vi "orc-red-threshing.vi"(5 "Blue or Luma or Val or Inten Range":cluster{"Lower value":i32, "Upper value":i32}={"Lower value"=0, "Upper value"=255}, 7 "Green or Sat Range":cluster{"Lower value":i32, "Upper value":i32}={"Lower value"=93, "Upper value"=255}, 9 "Red or Hue Range":cluster{"Lower value":i32, "Upper value":i32}={"Lower value"=6, "Upper value"=11}, 10 "Cluster":cluster{"Min Radius":sgl, "Max Radius":sgl}={"Min Radius"=10.0, "Max Radius"=100.0}, 11 "Image Src":T2, 13 "error in (no error)":errorcluster) -> (0 "Image Out":T2(plugin-control), 4 "Circles Data (calibrated)":T1(array[cluster]), 8 "Nb Circles":i32, 15 "error out":errorcluster)   [LabVIEW 2009]
uses:
  <vilib>/vision/Image Controls.llb/IMAQ Image.ctl
  <vilib>/vision/NI_Vision_Development_Module.lvlib
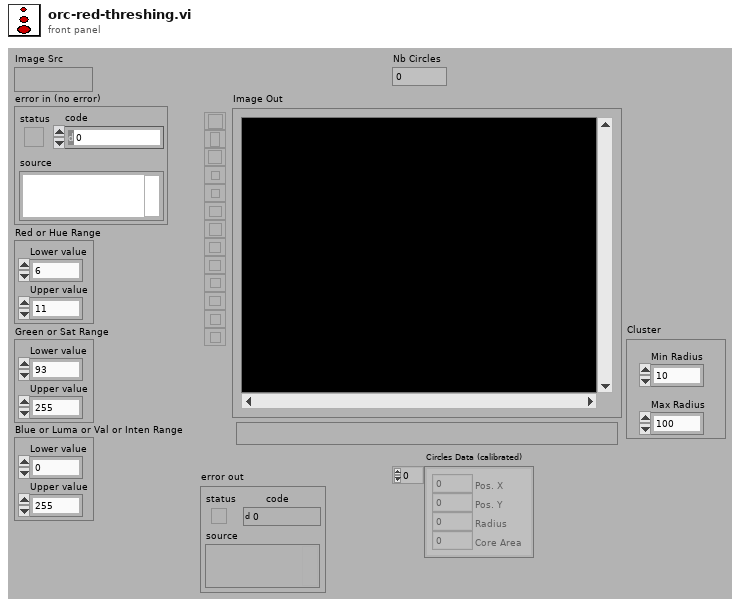
[diagram p1: front panel]
types:
  T1 = cluster{"Pos. X":i32, "Pos. Y":i32, "Radius":i32, "Core Area":i32}[]
  T2 = typedef "IMAQ Image.ctl" = refnum<image>
  T3 = enum32{"AutoM", "Close", "Dilate", "Erode", "Gradient", "Gradient out", "Gradient in", "Hit miss", "Open", "PClose", "POpen", "Thick", "Thin"}
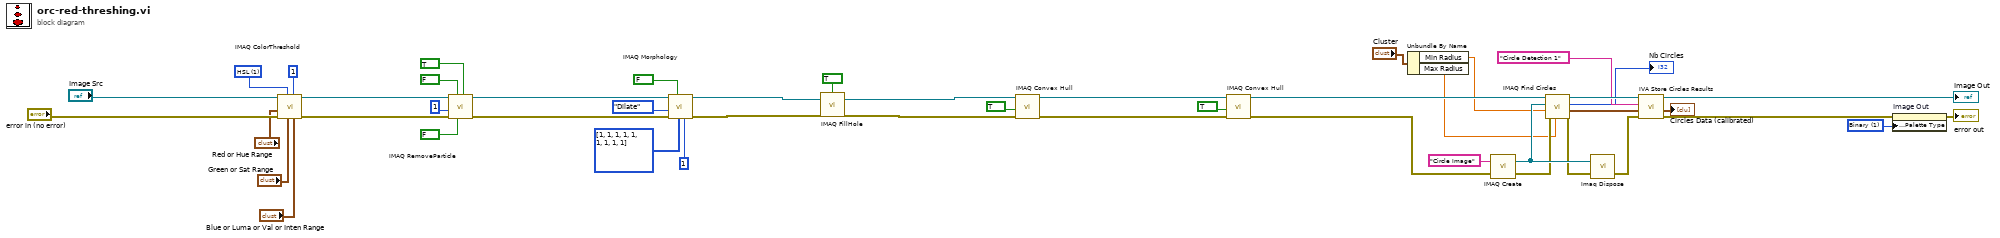
[diagram p0: block diagram]
diagram:
  w9 = u32 1 items=["Grayscale", "Binary", "Gradient", "Rainbow", "Temperature", "User Defined"] ("Palette")
  w44 = u16 1 items=["RGB", "HSL", "HSV", "HSI"] ("Color Mode")
  n1 = call "IMAQ ColorThreshold"("Blue or Luma or Val or Inten Range"="Blue or Luma or Val or Inten Range", "Replace Value"=1, "Green or Sat Range"="Green or Sat Range", "Color Mode"=w44, "error in (no error)"="error in (no error)", "Red or Hue Range"="Red or Hue Range", "Image Src"="Image Src") -> ("error out"=w41:errorcluster, "Image Dst Out"=w36:T2)  [unwired: 1 in, 2 out]
  n2 = call "IMAQ RemoveParticle"("Connectivity 4/8 (8)"=TRUE, "Low Pass/High Pass (Low)"=FALSE, "Square/Hexa (Square)"=FALSE, "error in (no error)"=w41, "Number of Erosion"=1, "Image Src"=w36) -> ("error out"=w35:errorcluster, "Image Dst Out"=w30:T2)  [unwired: 1 in, 3 out]
  n3 = call "IMAQ Morphology"("Number of iterations (1)"=1, "Structuring Element"=i32[][] [[1, 1, 1], [1, 1, 1], [1, 1, 1]], "Square/Hexa (Square)"=FALSE, "error in (no error)"=w35, "Operation"=T3."Dilate", "Image Src"=w30) -> ("error out"=w29:errorcluster, "Image Dst Out"=w27:T2)  [unwired: 1 in, 3 out]
  n4 = call "IMAQ FillHole"("error in (no error)"=w29, "Image Src"=w27, "Connectivity 4/8 (8)"=TRUE) -> ("error out"=w26:errorcluster, "Image Dst Out"=w25:T2)  [unwired: 1 in, 2 out]
  n5 = call "IMAQ Convex Hull"("error in (no error)"=w26, "Connectivity 4/8 (8)"=TRUE, "Image Src"=w25) -> ("error out"=w23:errorcluster, "Image Dst Out"=w22:T2)  [unwired: 1 in, 6 out]
  n6 = call "IMAQ Convex Hull"("error in (no error)"=w23, "Connectivity 4/8 (8)"=TRUE, "Image Src"=w22) -> ("error out"=w20:errorcluster, "Image Dst Out"=w13:T2)  [unwired: 1 in, 6 out]
  n7 = Unbundle By Name("Cluster") -> ("Min Radius"=w4:sgl, "Max Radius"=w3:sgl)
  n8 = call "IMAQ Create"("Image Name"="Circle Image", "error in (no error)"=w20) -> ("New Image"=w18:T2, "error out"=w17:errorcluster)  [unwired: 2 in, 1 out]
  n9 = call "IMAQ Find Circles"("Max Radius"=w3, "error in (no error)"=w17, "Min Radius"=w4, "Image Dst"=w18, "Image Src"=w13) -> ("error out"=w16:errorcluster, "Circles Data"=w11:T1, "Nb Circles"=→"Nb Circles":i32)  [unwired: 4 out]
  n10 = call "Imaq Dispose"("Image"=w18, "error in (no error)"=w16) -> ("error out"=w15:errorcluster)  [unwired: 1 in, 3 out]
  n11 = call <vilib>:"IVA Store Circles Results.vi"("error in (no error)"=w15, "Circles Data"=w11, "Step Name"="Circle Detection 1", "Image in"=w13) -> ("error out"=w14:errorcluster, "Circles Data (calibrated)"=→"Circles Data (calibrated)":T1, "Image dup"=→"Image Out":T2)  [unwired: 5 out]
  n12 = property on="Image Out" class="ImageControl"(error in=w14, "Palette:Palette Type"=w9) -> (error out=→"error out":errorcluster)  [unwired: 1 in, 1 out]
